vi "getModbusSubnetE.vi"(11 "Model in":refnum<class "Model.lvclass">) -> (2 "Modbus":refnum<class "IModbus.lvclass">, 3 "Model out":refnum<class "Model.lvclass">)   [LabVIEW 2016, in "Model.lvclass"]
uses:
  Model.lvclass
  Common_RT_Modbus/IModbus/IModbus.lvclass
  Model.lvclass/Model.ctl
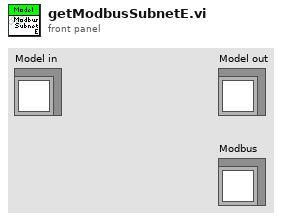
[diagram p1: front panel]
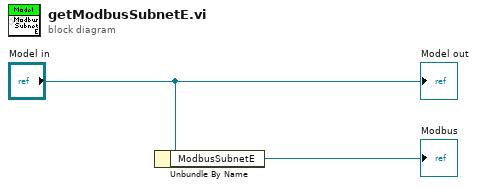
[diagram p0: block diagram]
diagram:
  n1 = Unbundle By Name("Model in") -> ("ModbusSubnetE"=→"Modbus":refnum<class "IModbus.lvclass">)
  "Model out" <- "Model in"
